vi "Test Comm.vi"() -> ()   [LabVIEW 2021]
uses:
  ChannelCommon/typedef/FIFO Config.ctl
  ChannelCommon/ChannelCommon.lvlib
  ChannelCommon/typedef/Datatype CAN.ctl
  CIFChannels/Typedef/Direction.ctl
  CIFChannels/CIFChannels.lvclass
  CIF_NIChn_FifoCAN.lvclass
  ChannelCommon/typedef/TimeStamps.ctl
panel:
  out "status":string
  out "pass":bool
  out "error out":errorcluster
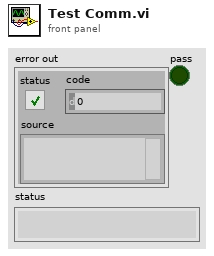
[diagram p1: front panel]
types:
  T1 = typedef "CIFChannels.lvclass/Direction.ctl" = enum16{"Publisher", "Subscriber"}
  T2 = typedef "ChannelCommon.lvlib/TimeStamps.ctl" = cluster{"ClockID":u8, "T0":u64, "T_Out":u64}
  T3 = typedef "ChannelCommon.lvlib/Datatype CAN.ctl" = cluster{"payload":u8[], "identifier":u32, "Tags":u8, "Timestamp":u64}
  T4 = typedef "ChannelCommon.lvlib/FIFO Config.ctl" = cluster{"Depth":u64, "Flags":u64, "ClockID":u8}
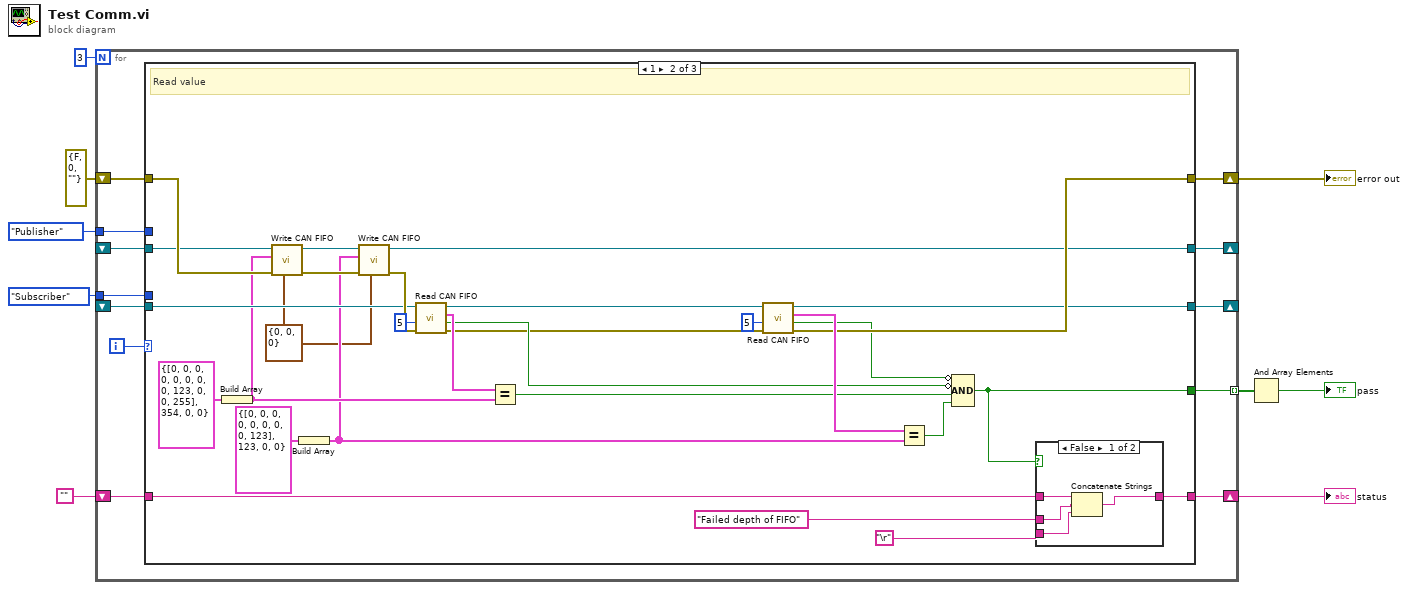
[diagram p0: block diagram]
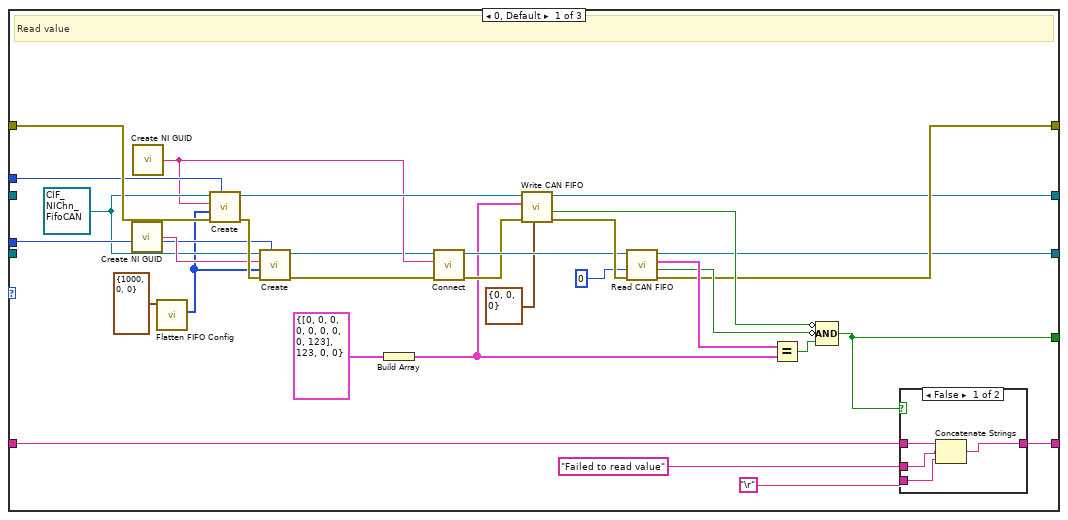
[diagram p2: hidden frame]
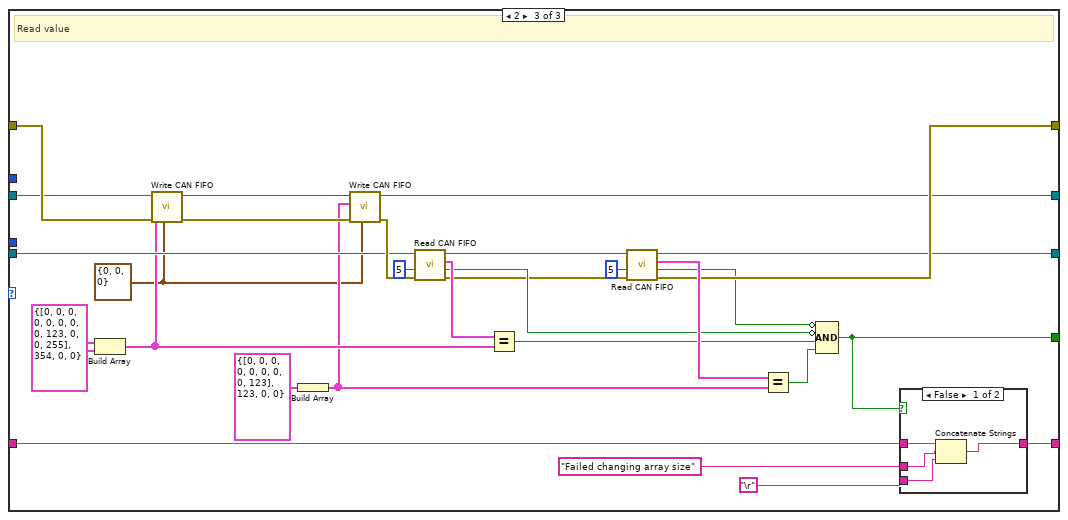
[diagram p5: hidden frame]
diagram:
  n1 = for {
    N: 3 -> [_]
    tunnel: [w21] -> w9 mode=indexing
    shift-right: [w19] -> w4
    shift-left: errorcluster {"status"=FALSE, "code"=0, "source"=""} ("error out") -> [w20]
    shift-right: [w16] -> w5
    shift-left: "" -> [w17]
    tunnel: Direction."Subscriber" ("Direction") -> [w15]
    tunnel: Direction."Publisher" ("Direction") -> [w14]
    shift-right: [w13] -> _
    shift-left: _ -> [w10]
    shift-right: [w12] -> _
    shift-left: _ -> [w11]
    i -> [w18]
    n2 = case shown="1" w18 {
      tunnel: [w47 w81 w114] -> w21
      tunnel: w20 -> [w45 w75 w108]
      tunnel: [w28 w79 w112] -> w19
      tunnel: w17 -> [w52 w85 w118]
      tunnel: [w51 w84 w117] -> w16
      tunnel: w15 -> [w43 _ _]
      tunnel: w14 -> [w42 _ _]
      tunnel: [w26 w78 w111] -> w13
      tunnel: [w25 w77 w110] -> w12
      tunnel: w11 -> [_ w62 w96]
      tunnel: w10 -> [_ w63 w97]
      frame 0, Default {
        w41 = refnum<class "CIF_NIChn_FifoCAN.lvclass"> refnum ("CIF_NIChn_FifoCAN.lvclass")
        # "Read value"
        n3 = call <vilib>:"Create NI GUID.vi"() -> ("NI GUID"=w44:string)
        n4 = call <vilib>:"Create NI GUID.vi"() -> ("NI GUID"=w32:string)
        n5 = call "Flatten FIFO Config.vi"("FIFO Config in"=T4 {"Depth"=1000, "Flags"=0, "ClockID"=0}) -> ("Flattened Data out"=w39:u8[])  [unwired: 8 in, 2 out]
        n6 = call-dynamic "Create.vi"("Direction"=w42, "error in (no error)"=w45, "Custom Config Data"=w39, "Name"=w32, "CIFTag in"=w41) -> ("error out"=w46:errorcluster, "CIFTag out"=w38:refnum<class "CIF_NIChn_FifoCAN.lvclass">)  [unwired: 5 in]
        n7 = call-dynamic "Create.vi"("Direction"=w43, "error in (no error)"=w46, "Custom Config Data"=w39, "Name"=w44, "CIFTag in"=w41) -> ("error out"=w31:errorcluster, "CIFTag out"=w29:refnum<class "CIF_NIChn_FifoCAN.lvclass">)  [unwired: 5 in]
        n8 = Build Array(T3 {"payload"=[0, 0, 0, 0, 0, 0, 0, 0, 123], "identifier"=123, "Tags"=0, "Timestamp"=0} ("Data")) -> (w23:T3[])
        n9 = call-dynamic "Connect.vi"("error in (no error)"=w31, "Connection Name"=w32, "CIFTag in"=w29) -> ("error out"=w30:errorcluster, "CIFTag out"=w33:refnum<class "CIF_NIChn_FifoCAN.lvclass">)  [unwired: 7 in]
        n10 = call-dynamic "Write CAN FIFO.vi"("FIFO Timestamps"=T2 {"ClockID"=0, "T0"=0, "T_Out"=0}, "error in (no error)"=w30, "Data"=w23, "CIFTag in"=w38) -> ("error out"=w37:errorcluster, "timed out?"=w35:bool, "CIFTag out"=w25:refnum<class "CIF_NIChn_FifoCAN.lvclass">)  [unwired: 5 in]
        n11 = call-dynamic "Read CAN FIFO.vi"("error in (no error)"=w37, "Timeout (ms)"=0, "CIFTag in"=w33) -> ("error out"=w28:errorcluster, "timed out?"=w34:bool, "Data"=w36:T3[], "CIFTag out"=w26:refnum<class "CIF_NIChn_FifoCAN.lvclass">)  [unwired: 4 in, 1 out]
        n12 = Equal?(x=w36, y=w23) -> (x = y?=w48:bool)
        n13 = Compound Arithmetic op=AND(invert w35, invert w34, w48) -> (w47:bool)
        n14 = case shown="False" w47 {
          tunnel: w52 -> [w56 w57]
          tunnel: [w53 w57] -> w51
          tunnel: "Failed to read value" -> [w55 _]
          tunnel: "\r" -> [w54 _]
          frame False {
            n15 = Concatenate Strings(w56, w55, w54) -> (w53:string)
          }
          frame True {
          }
        }
      }
      frame 1 {
        w58 = T2 {"ClockID"=0, "T0"=0, "T_Out"=0} ("FIFO Timestamps")
        # "Read value"
        n16 = Build Array(T3 {"payload"=[0, 0, 0, 0, 0, 0, 0, 0, 123, 0, 0, 255], "identifier"=354, "Tags"=0, "Timestamp"=0} ("Data")) -> (w61:T3[])
        n17 = call-dynamic "Write CAN FIFO.vi"("FIFO Timestamps"=w58, "error in (no error)"=w75, "Data"=w61, "CIFTag in"=w62) -> ("error out"=w68:errorcluster, "CIFTag out"=w76:refnum<class "CIF_NIChn_FifoCAN.lvclass">)  [unwired: 5 in, 1 out]
        n18 = Build Array(T3 {"payload"=[0, 0, 0, 0, 0, 0, 0, 0, 123], "identifier"=123, "Tags"=0, "Timestamp"=0} ("Data")) -> (w59:T3[])
        n19 = call-dynamic "Write CAN FIFO.vi"("FIFO Timestamps"=w58, "error in (no error)"=w68, "Data"=w59, "CIFTag in"=w76) -> ("CIFTag out"=w77:refnum<class "CIF_NIChn_FifoCAN.lvclass">)  [unwired: 5 in, 2 out]
        n20 = call-dynamic "Read CAN FIFO.vi"("error in (no error)"=w68, "Timeout (ms)"=5, "CIFTag in"=w63) -> ("error out"=w67:errorcluster, "timed out?"=w69:bool, "Data"=w74:T3[], "CIFTag out"=w66:refnum<class "CIF_NIChn_FifoCAN.lvclass">)  [unwired: 4 in, 1 out]
        n21 = Equal?(x=w74, y=w61) -> (x = y?=w71:bool)
        n22 = call-dynamic "Read CAN FIFO.vi"("error in (no error)"=w67, "Timeout (ms)"=5, "CIFTag in"=w66) -> ("error out"=w79:errorcluster, "timed out?"=w70:bool, "Data"=w80:T3[], "CIFTag out"=w78:refnum<class "CIF_NIChn_FifoCAN.lvclass">)  [unwired: 4 in, 1 out]
        n23 = Equal?(x=w80, y=w59) -> (x = y?=w72:bool)
        n24 = Compound Arithmetic op=AND(invert w70, invert w69, w71, w72) -> (w81:bool)
        n25 = case shown="False" w81 {
          tunnel: w85 -> [w89 w90]
          tunnel: [w86 w90] -> w84
          tunnel: "Failed depth of FIFO" -> [w88 _]
          tunnel: "\r" -> [w87 _]
          frame False {
            n26 = Concatenate Strings(w89, w88, w87) -> (w86:string)
          }
          frame True {
          }
        }
      }
      frame 2 {
        w91 = T2 {"ClockID"=0, "T0"=0, "T_Out"=0} ("FIFO Timestamps")
        w92 = T3 {"payload"=[0, 0, 0, 0, 0, 0, 0, 0, 123, 0, 0, 255], "identifier"=354, "Tags"=0, "Timestamp"=0} ("Data")
        # "Read value"
        n27 = Build Array(w92, w92) -> (w95:T3[])
        n28 = call-dynamic "Write CAN FIFO.vi"("FIFO Timestamps"=w91, "error in (no error)"=w108, "Data"=w95, "CIFTag in"=w96) -> ("error out"=w102:errorcluster, "CIFTag out"=w109:refnum<class "CIF_NIChn_FifoCAN.lvclass">)  [unwired: 5 in, 1 out]
        n29 = Build Array(T3 {"payload"=[0, 0, 0, 0, 0, 0, 0, 0, 123], "identifier"=123, "Tags"=0, "Timestamp"=0} ("Data")) -> (w94:T3[])
        n30 = call-dynamic "Write CAN FIFO.vi"("FIFO Timestamps"=w91, "error in (no error)"=w102, "Data"=w94, "CIFTag in"=w109) -> ("CIFTag out"=w110:refnum<class "CIF_NIChn_FifoCAN.lvclass">)  [unwired: 5 in, 2 out]
        n31 = call-dynamic "Read CAN FIFO.vi"("error in (no error)"=w102, "Timeout (ms)"=5, "CIFTag in"=w97) -> ("error out"=w101:errorcluster, "timed out?"=w103:bool, "Data"=w107:T3[], "CIFTag out"=w100:refnum<class "CIF_NIChn_FifoCAN.lvclass">)  [unwired: 4 in, 1 out]
        n32 = Equal?(x=w107, y=w95) -> (x = y?=w105:bool)
        n33 = call-dynamic "Read CAN FIFO.vi"("error in (no error)"=w101, "Timeout (ms)"=5, "CIFTag in"=w100) -> ("error out"=w112:errorcluster, "timed out?"=w104:bool, "Data"=w113:T3[], "CIFTag out"=w111:refnum<class "CIF_NIChn_FifoCAN.lvclass">)  [unwired: 4 in, 1 out]
        n34 = Equal?(x=w113, y=w94) -> (x = y?=w106:bool)
        n35 = Compound Arithmetic op=AND(invert w104, invert w103, w105, w106) -> (w114:bool)
        n36 = case shown="False" w114 {
          tunnel: w118 -> [w122 w123]
          tunnel: [w119 w123] -> w117
          tunnel: "Failed changing array size" -> [w121 _]
          tunnel: "\r" -> [w120 _]
          frame False {
            n37 = Concatenate Strings(w122, w121, w120) -> (w119:string)
          }
          frame True {
          }
        }
      }
    }
  }
  "error out" <- w4
  "status" <- w5
  n38 = And Array Elements(Boolean array=w9) -> (logical AND=→"pass":bool)
